vi "Write Boolean.vi"(8 "error in (no error)":errorcluster, 9 "value":bool, 10 "Tag Name":string, 11 "Current Value Table in":refnum<class "Current Value Table.lvclass">) -> (0 "error out":errorcluster, 3 "Current Value Table out":refnum<class "Current Value Table.lvclass">)   [LabVIEW 2024, in "Current Value Table.lvlib" / "Current Value Table.lvclass"]
uses:
  Current Value Table.lvclass
  Get Boolean Notifier Ref.vi
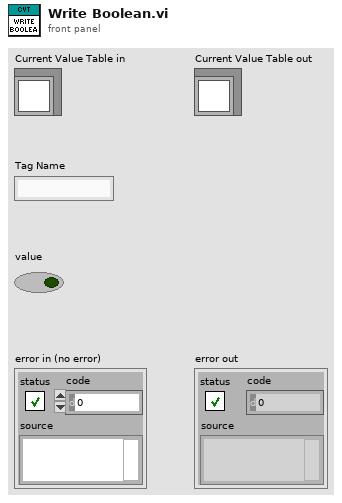
[diagram p1: front panel]
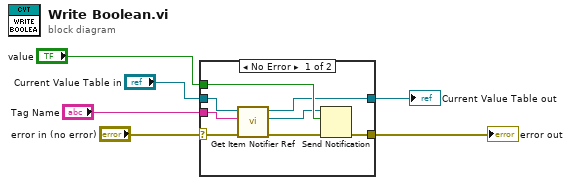
[diagram p0: block diagram]
diagram:
  n1 = case shown="No Error" "error in (no error)" {
    selector: "error in (no error)" -> [w9 w16]
    tunnel: [w13 w16] -> w5
    tunnel: [w7 w15] -> w3
    tunnel: "Current Value Table in" -> [w12 w15]
    tunnel: "Tag Name" -> [w8 _]
    tunnel: "value" -> [w14 _]
    frame No Error {
      n2 = call-poly "Get Item Notifier Ref.vi"("error in (no error)"=w9, "Tag Name"=w8, "Current Value Table in"=w12) -> ("error out"=w10:errorcluster, "notifier out"=w11:refnum<notifier>, "Current Value Table out"=w7:refnum<class "Current Value Table.lvclass">)  [unwired: 6 in]
      n3 = Send Notification(notification=w14, notifier=w11, error in (no error)=w10) -> (error out=w13:errorcluster)  [unwired: 1 out]
    }
    frame Error {
    }
  }
  "error out" <- w5
  "Current Value Table out" <- w3
